vi "LV SciSDK LIST STOP.vi"(8 "error in (no error)":errorcluster, 9 "Board Handle In":T1, 10 "List Handle In":cluster{"List Path":string, "List Name":string}) -> (0 "error out":errorcluster, 1 "Board Handle Out":T1, 2 "List Handle Out":cluster{"List Path":string, "List Name":string}, 3 "NI Error Code":i32)   [LabVIEW 2021, in "SciSDK_Labview.lvlib"]
doc: "You need this VI to execute list stop command"
uses:
  SciSDK_Labview.lvlib
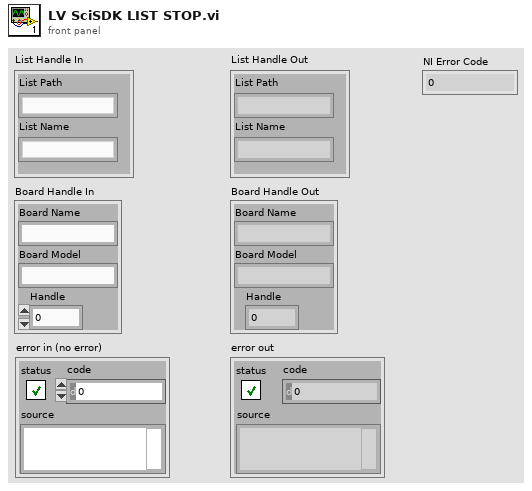
[diagram p1: front panel]
types:
  T1 = cluster{"Board Name":string, "Board Model":string, "Handle":u64}
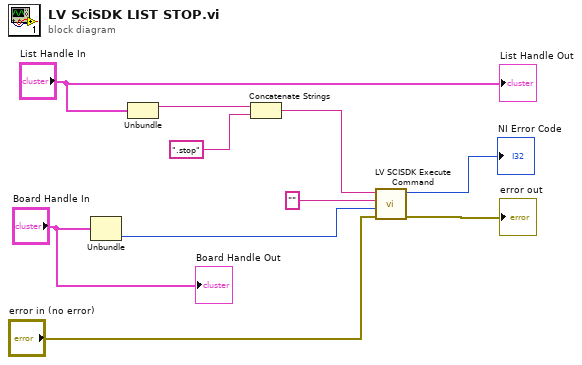
[diagram p0: block diagram]
diagram:
  n1 = Unbundle("Board Handle In") -> ("Handle"=w1:u64)  [unwired: 2 out]
  n2 = Unbundle("List Handle In") -> ("List Path"=w3:string)  [unwired: 1 out]
  n3 = Concatenate Strings(w3, ".stop" ("string")) -> (w8:string)
  n4 = call "LV SCISDK Execute Command.vi"("error in (no error)"="error in (no error)", "handle"=w1, "value"="", "Path"=w8) -> ("error out"=→"error out":errorcluster, "function return"=→"NI Error Code":i32)  [unwired: 5 in, 1 out]
  "List Handle Out" <- "List Handle In"
  "Board Handle Out" <- "Board Handle In"
